vi "lib_QMH_Admin Class--control.vi"() -> ()   [LabVIEW 2018, in "lib_QMH_Module_Admin.lvclass"]
uses:
  lib_QMH_Module_Admin.lvclass
panel:
  in  "Module Admin":refnum<class "lib_QMH_Module_Admin.lvclass">
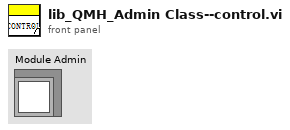
[diagram p1: front panel]
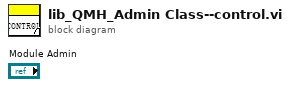
[diagram p0: block diagram]
diagram:
